vi "Remove From Subpanel.vi"(8 "error in (no error)":errorcluster, 11 "Actor API in":refnum<class "Actor API.lvclass">) -> (0 "error out":errorcluster)   [LabVIEW 2015, in "Actor API.lvclass"]
uses:
  Actor API.lvclass
  Messaging/Message/Message.lvclass/Message.ctl
  Messaging/Message/Message.lvclass
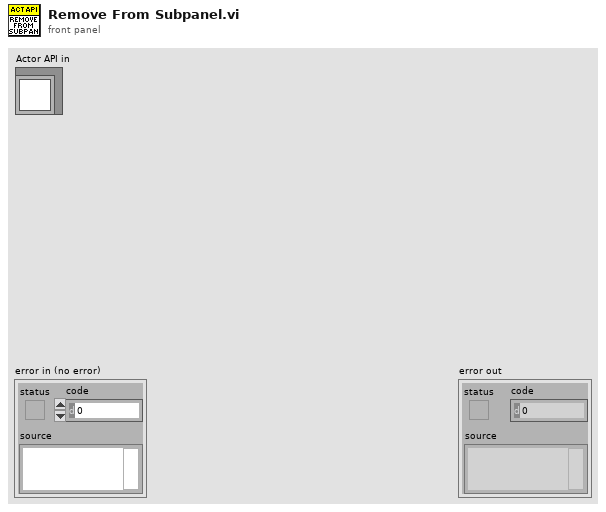
[diagram p1: front panel]
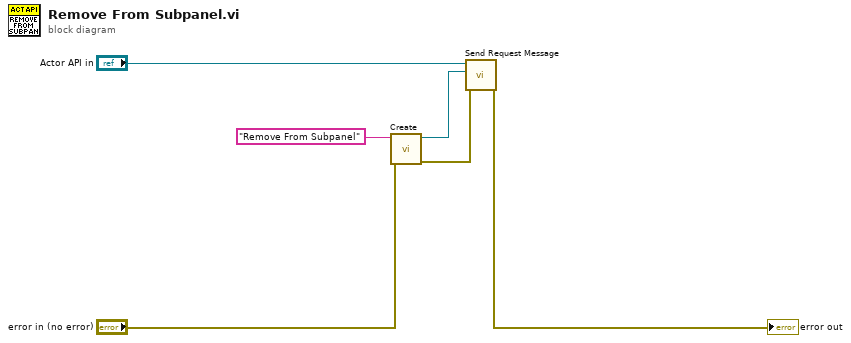
[diagram p0: block diagram]
diagram:
  n1 = call "Create.vi"("error in (no error)"="error in (no error)", "Name"="Remove From Subpanel" ("format string")) -> ("error out"=w2:errorcluster, "Message out"=w1:refnum<class "Message.lvclass">)  [unwired: 8 in]
  n2 = call-dynamic "Send Request Message.vi"("error in (no error)"=w2, "Message"=w1, "Actor API in"="Actor API in") -> ("error out"=→"error out":errorcluster)  [unwired: 8 in]
